vi "Pop Up After.vi"(10 "mode":T1) -> ()   [LabVIEW 2019, in "LSS.lvlib"]
doc: "Pop up dialog from the example done using LSS.\n\n<b>Inputs:</b>\n<b>mode</b> - Used to select between different styles available for the pop up dialog."
uses:
  LSS.lvlib
  Themes.ctl
  <vilib>/Utility/miscctls.llb/LVBoundsTypeDef.ctl
panel:
  in  "Button4":bool
  in  "Button3":bool
  in  "Button2":bool
  in  "Button1":bool
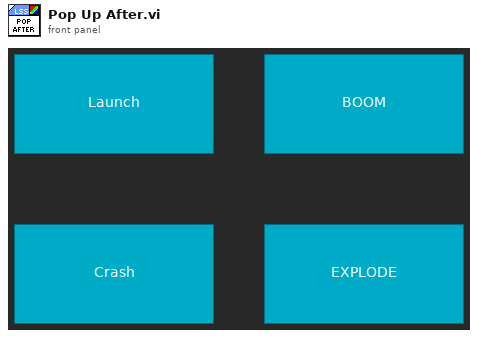
[diagram p1: front panel]
types:
  T1 = typedef "LSS.lvlib/Themes.ctl" = enum16{"SPACE", "ATK", "THEME1", "THEME2"}
  T2 = typedef "LVBoundsTypeDef.ctl" = cluster{"Width":u32, "Height":u32}
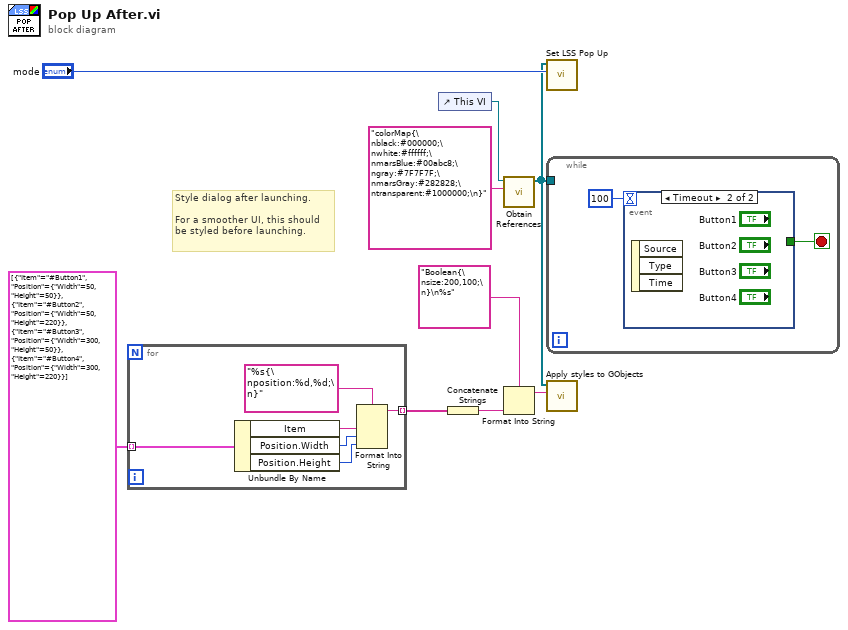
[diagram p0: block diagram]
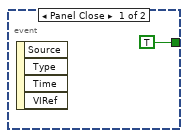
[diagram p2: hidden frame]
diagram:
  # "Style dialog after launching.\n\nFor a smoother UI, this should\nbe styled before launching."
  n1 = for {
    tunnel: cluster{"Item":string, "Position":T2}[] [{"Item"="#Button1", "Position"={"Width"=50, "Height"=50}}, {"Item"="#Button2", "Position"={"Width"=50, "Height"=220}}, {"Item"="#Button3", "Position"={"Width"=300, "Height"=50}}, {"Item"="#Button4", "Position"={"Width"=300, "Height"=220}}] -> [w15] mode=indexing
    tunnel: [w10] -> w5 mode=indexing
    n2 = Unbundle By Name(w15) -> ("Item"=w13:string, "Position.Width"=w12:u32, "Position.Height"=w11:u32)
    n3 = Format Into String(format string="%s{\nposition:%d,%d;\n}", w13, w12, w11) -> (resulting string=w10:string)  [unwired: 2 in, 1 out]
  }
  n4 = control-ref of="This VI"() -> (w9:refnum<vi>)
  n5 = Concatenate Strings(w5) -> (w3:string)
  n6 = call "Obtain References.vi"("colorMap"="colorMap{\nblack:#000000;\nwhite:#ffffff;\nmarsBlue:#00abc8;\ngray:#7F7F7F;\nmarsGray:#282828;\ntransparent:#1000000;\n}", "VI in"=w9) -> ("Front Panel Objects"=w1:refnum<vi>[])  [unwired: 8 in, 1 out]
  n7 = Format Into String(format string="Boolean{\nsize:200,100;\n}\n%s" ("String"), w3) -> (resulting string=w2:string)  [unwired: 2 in, 1 out]
  n8 = call "Set LSS Pop Up.vi"("Theme Choice"="mode", "Front Panel Objects"=w1) -> ()  [unwired: 10 in]
  n9 = while {
    tunnel: w1 -> [_]
    stop <- w16 stop-if-true
    n10 = event shown="[1] Timeout" {
      selector: _ -> [_ _]
      dyn-events: _ -> [_ _]
      timeout: 100 -> [_ _]
      tunnel: [TRUE _] -> w16
      event Panel Close {
        n11 = event-data() -> ()  [unwired: 1 in, 4 out]
      }
      event Timeout {
        n12 = event-data() -> ()  [unwired: 1 in, 3 out]
      }
    }
  }
  n13 = call "Apply styles to GObjects.vi"("Style Sheet"=w2, "Front Panel Objects"=w1) -> ()  [unwired: 8 in, 2 out]
